vi "Configure Serial Output Channels.vi"(0 "fpga interface in":refnum<k20>, 1 "start trigger delay (s)":dbl, 5 "serial output channels":string[](array[string]), 7 "source file paths":T2[](array[typedef]), 9 "dram partition sizes (bytes)":u64[](array[numeric]), 11 "error in (no error)":errorcluster, 12 "packet timing error threshold (s)":dbl=1e-06 format="%#_6p", 13 "fpga buffer start thresholds":T1={"timestamp buffer start threshold"=1023, "packet data buffer start threshold (bytes)"=32768, "dram partition start threshold (bytes)"=2147483648}, 14 "enable i2c tap (all channels)":bool=TRUE) -> (4 "fpga interface out":refnum<k20>, 15 "error out":errorcluster)   [LabVIEW 2023, in "GettingStarted_Gen_148X_Host.lvlib"]
uses:
  GettingStarted_Gen_148X_Host.lvlib
  Types/Channel Source File Paths.ctl
  Types/FPGA Buffer Start Thresholds.ctl
  FPGA/Gen/Types/Serial Output Channel Datapath Configuration.ctl
  Types/148x_Gen_FPGA_Reference.ctl
  e175faef-8d0e-4f24-ae54-e9c9e67f6f95.vi
  <vilib>/rvi/errors/niLvFpgaAdjustHostInterfaceError.vi
  <vilib>/rvi/interface/nirviReadWriteControl/nirviReadWriteControl.xnode
  FPGA/Gen/GettingStarted_Gen_148X_FPGA.lvlib
  <instrlib>/FlexRIO/Automotive Vision Utility/v1/Host/Automotive Vision Utility.lvlib
  NiFpgaLv.dll
  <vilib>/rvi/interface/Simulation/niFpgaSimulationCallBeginRW.vi
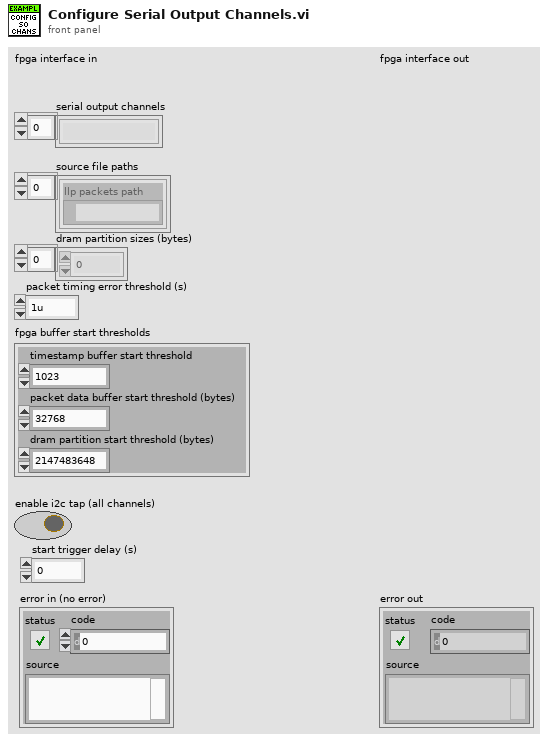
[diagram p1: front panel]
types:
  T1 = typedef "GettingStarted_Gen_148X_Host.lvlib/FPGA Buffer Start Thresholds.ctl" = cluster{"timestamp buffer start threshold":u32, "packet data buffer start threshold (bytes)":u64, "dram partition start threshold (bytes)":u64}
  T2 = typedef "GettingStarted_Gen_148X_Host.lvlib/Channel Source File Paths.ctl" = cluster{"llp packets path":path}
  T3 = typedef "GettingStarted_Gen_148X_Host.lvlib/148x_Gen_FPGA_Reference.ctl" = refnum<k20>
  T4 = typedef "GettingStarted_Gen_148X_FPGA.lvlib/Serial Output Channel Datapath Configuration.ctl" = cluster{"dram flush threshold (bytes)":u64, "packet data buffer fill threshold (bytes)":u64, "timestamp buffer fill threshold":u32, "packet timing error threshold (cycles)":u64, "channel enabled":bool, "dram partition fill threshold (bytes)":u64, "enable i2c tap bridge":bool, "packet timestamp offset (cycles)":i64}
  T5 = typedef "Automotive Vision Utility.lvlib/Serial Channel Type.ctl" = enum16{"Serial Input Channel", "Serial Output Channel", "Unknown Channel Type"}
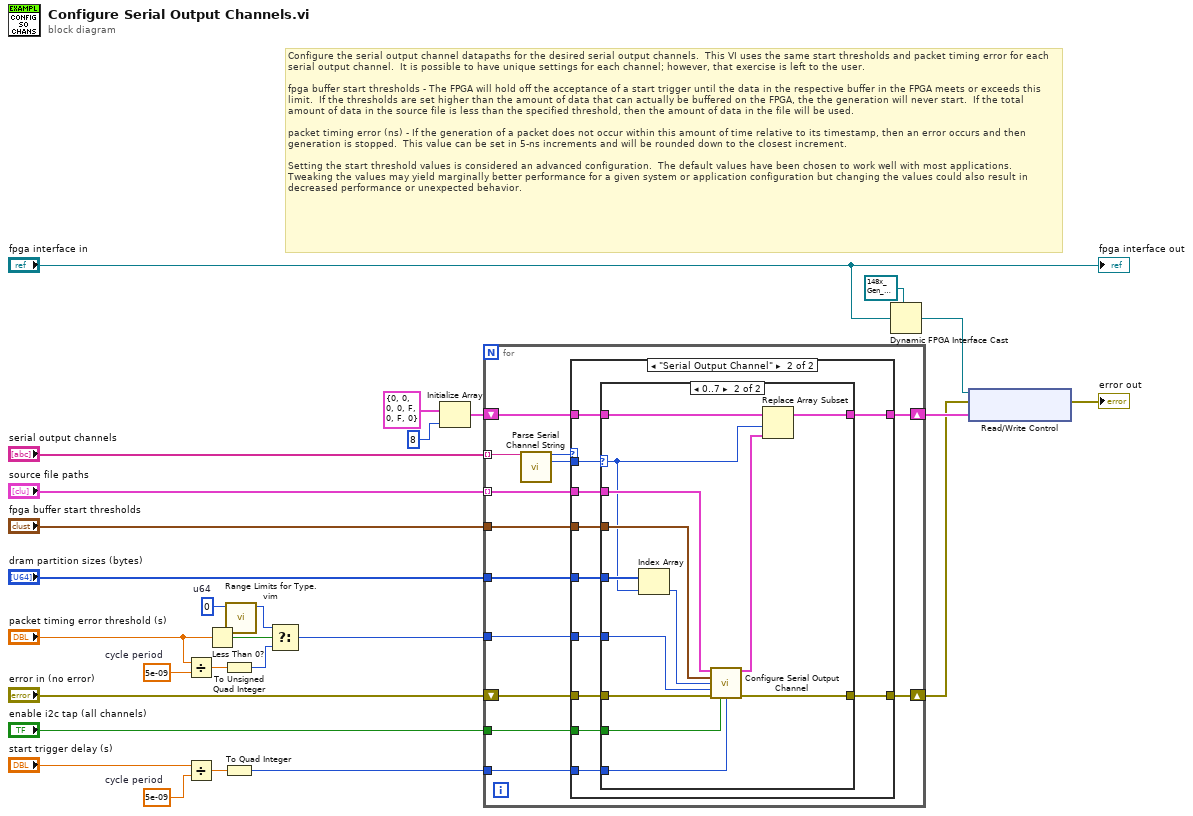
[diagram p0: block diagram]
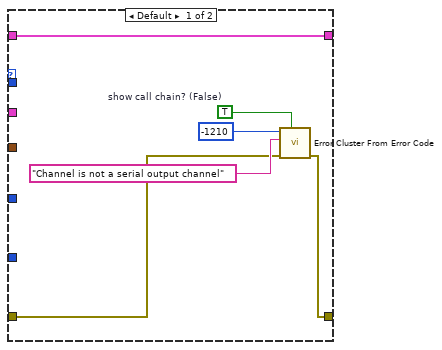
[diagram p2: hidden frame]
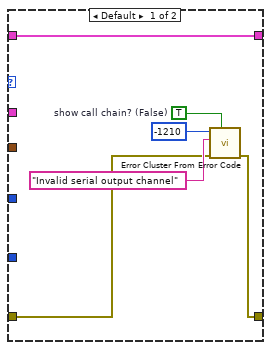
[diagram p3: hidden frame]
diagram:
  w1 = 5e-09  # cycle period
  w9 = 5e-09  # cycle period
  w10 = u64 0  # u64
  # "Configure the serial output channel datapaths for the desired serial output channels.  This VI uses the same start thresholds and packet timing error for each serial output channel.  It is possible to have unique settings for each channel; however, that exercise is left to the user.\n\nfpga buffer start thresholds - The FPGA will hold off the acceptance of a start trigger until the data in the respective buffer in the FPGA meets or exceeds this limit.  If the thresholds are set higher than the amount of data that can actually be buffered on the FPGA, the the generation will never start.  If the total amount of data in the source file is less than the specified threshold, then the amount of data in the file will be used.  \n\npacket timing error (ns) - If the generation of a packet does not occur within this amount of time relative to its timestamp, then an error occurs and then generation is stopped.  This value can be set in 5-ns increments and will be rounded down to the closest increment.\n\nSetting the start threshold values is considered an advanced configuration.  The default values have been chosen to work well with most applications.  Tweaking the values may yield marginally better performance for a given system or application configuration but changing the values could also result in decreased performance or unexpected behavior."
  n1 = Divide(x="packet timing error threshold (s)", y=w9) -> (x/y=w13:dbl)
  n2 = Divide(x="start trigger delay (s)", y=w1) -> (x/y=w4:dbl)
  n3 = Less Than 0?(x="packet timing error threshold (s)") -> (x < 0?=w15:bool)
  n4 = To Unsigned Quad Integer(1:w13) -> (0:w12:u64)
  n5 = To Quad Integer(1:w4) -> (0:w3:i64)
  n6 = call "Range Limits for Type.vim"("type"=w10) -> ("maximum value for type"=w11:u64)  [unwired: 9 in, 1 out]
  n7 = Select(t=w11, s=w15, f=w12) -> (s? t:f=w14:u64)
  n8 = Initialize Array(T4 {"dram flush threshold (bytes)"=0, "packet data buffer fill threshold (bytes)"=0, "timestamp buffer fill threshold"=0, "packet timing error threshold (cycles)"=0, "channel enabled"=FALSE, "dram partition fill threshold (bytes)"=0, "enable i2c tap bridge"=FALSE, "packet timestamp offset (cycles)"=0} ("datapath config"), 8 ("dimension size")) -> (w26:T4[])
  n9 = for {
    tunnel: "serial output channels" -> [w39] mode=indexing
    tunnel: "source file paths" -> [w38] mode=indexing
    shift-right: [w32] -> w18
    shift-left: w26 -> [w36]
    shift-right: [w35] -> w16
    shift-left: "error in (no error)" -> [w34]
    tunnel: w14 -> [w33]
    tunnel: "fpga buffer start thresholds" -> [w31]
    tunnel: "dram partition sizes (bytes)" -> [w30]
    tunnel: "enable i2c tap (all channels)" -> [w29]
    tunnel: w3 -> [w28]
    n10 = call <instrlib>:"Parse Serial Channel String.vi"("serial channel string"=w39) -> ("serial channel type"=w40:T5, "channel number"=w37:i32)  [unwired: 13 in]
    n11 = case shown="\"Serial Output Channel\"" w40 {
      tunnel: w38 -> [_ w57]
      tunnel: w37 -> [_ w51]
      tunnel: w36 -> [w46 w56]
      tunnel: [w41 w55] -> w35
      tunnel: w34 -> [w42 w54]
      tunnel: w33 -> [_ w53]
      tunnel: [w46 w52] -> w32
      tunnel: w31 -> [_ w50]
      tunnel: w30 -> [_ w49]
      tunnel: w29 -> [_ w48]
      tunnel: w28 -> [_ w47]
      frame Default {
        w43 = TRUE  # show call chain? (False)
        n12 = call <vilib>:"Error Cluster From Error Code.vi"("show call chain? (False)"=w43, "error in (no error)"=w42, "error message (\"\")"="Channel is not a serial output channel" ("error message (\"\")"), "error code (0)"=-1210) -> ("error out"=w41:errorcluster)  [unwired: 5 in]
      }
      frame "Serial Output Channel" {
        n13 = case shown="0..7" w51 {
          selector: w51 -> [_ w67]
          tunnel: w57 -> [_ w76]
          tunnel: w56 -> [w58 w75]
          tunnel: [w60 w73] -> w55
          tunnel: w54 -> [w59 w72]
          tunnel: w53 -> [_ w69]
          tunnel: [w58 w71] -> w52
          tunnel: w50 -> [_ w70]
          tunnel: w49 -> [_ w68]
          tunnel: w48 -> [_ w65]
          tunnel: w47 -> [_ w64]
          frame Default {
            w62 = TRUE  # show call chain? (False)
            n14 = call <vilib>:"Error Cluster From Error Code.vi"("show call chain? (False)"=w62, "error in (no error)"=w59, "error message (\"\")"="Invalid serial output channel" ("error message (\"\")"), "error code (0)"=-1210) -> ("error out"=w60:errorcluster)  [unwired: 5 in]
          }
          frame 0..7 {
            n15 = Index Array(array=w68, index=w67) -> (element=w66:u64)
            n16 = call "Configure Serial Output Channel.vi"("channel source file paths"=w76, "fpga buffer start thresholds"=w70, "dram partition size (bytes)"=w66, "packet timing error threshold (cycles)"=w69, "error in (no error)"=w72, "enable i2c tap (all channels)"=w65, "start trigger delay (cycles)"=w64) -> ("datapath config"=w74:T4, "error out"=w73:errorcluster)  [unwired: 7 in]
            n17 = Replace Array Subset(array=w75, new element=w74, index=w67) -> (w71:T4[])
          }
        }
      }
    }
  }
  n18 = Dynamic FPGA Interface Cast(Session In=T3 refnum ("FPGA VI Reference Out"), Type="fpga interface in") -> (Session Out=w19:T3)
  n19 = xnode "Read/Write Control"("FPGA VI Reference In"=w19, "error in"=w16, "channel configs"=w18) -> ("error out"=→"error out":errorcluster)  [unwired: 1 out]
  "fpga interface out" <- "fpga interface in"
